vi "CRC16.vi"(3 "Swap CRC16 Bytes?(T)":bool=TRUE, 4 "Data":string="\u0001\u0003\u0000\u0000\u0000\u0002") -> (0 "CRC":u16=50187 format="%x", 1 "Data+CRC16":string)   [LabVIEW 2017]
doc: "Computes the CRC-16 checksum of Data using polynomial 0xA001 and returns the checksum together with Data with the checksum appended. Set Swap CRC16 Bytes?(T) to FALSE to keep the checksum bytes in calculation order."
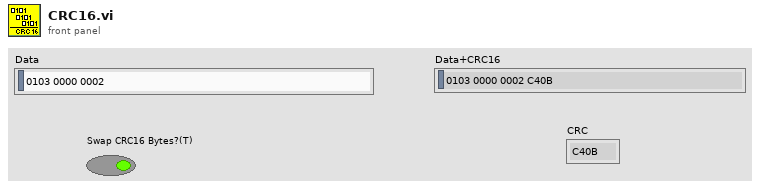
[diagram p1: front panel]
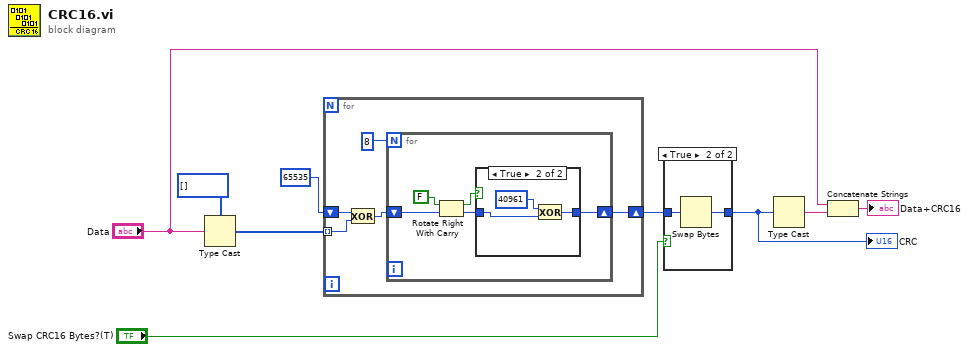
[diagram p0: block diagram]
diagram:
  n1 = Type Cast(type=u8[] [], x="Data") -> (*(type *) &x=w7:u8[])
  n2 = for {
    tunnel: w7 -> [w14] mode=indexing
    shift-right: [w11] -> w3
    shift-left: u16 65535 -> [w13]
    n3 = Exclusive Or(1:w14, 2:w13) -> (0:w12:u16)
    n4 = for {
      N: 8 -> [_]
      shift-right: [w15] -> w11
      shift-left: w12 -> [w19]
      n5 = Rotate Right With Carry(2:w19, 3:FALSE ("进位")) -> (0:w16:u16, 1:w17:bool)
      n6 = case shown="True" w17 {
        tunnel: w16 -> [w20 w23]
        tunnel: [w20 w21] -> w15
        frame False {
        }
        frame True {
          n7 = Exclusive Or(1:w23, 2:u16 40961) -> (0:w21:u16)
        }
      }
    }
  }
  n8 = case shown="True" "Swap CRC16 Bytes?(T)" {
    tunnel: [w24 w26] -> w6
    tunnel: w3 -> [w24 w25]
    frame False {
    }
    frame True {
      n9 = Swap Bytes(anything=w25) -> (byte swapped=w26:u16)
    }
  }
  "CRC" <- w6
  n10 = Type Cast(x=w6) -> (*(type *) &x=w5:string)  [unwired: 1 in]
  n11 = Concatenate Strings("Data", w5) -> (→"Data+CRC16":string)
